vi "Stimulus to 5734 Io Emulator.vi"() -> ()   [LabVIEW 2012]
panel:
  in  "Marker Position":u32
  in  "Frequency":dbl=10000000.0 format="%#_p"
  in  "signal type":T1(ring)
  in  "stop":bool
  out "Data Generated":cluster{"Data":i16, i16}(graph)
  in  "sampling info":cluster{"Fs":dbl, "#s":dbl}={"Fs"=250000000.0, "#s"=1000.0} {"Fs" format="%#_p"}
  # "You cannot change waveform type on the fly"
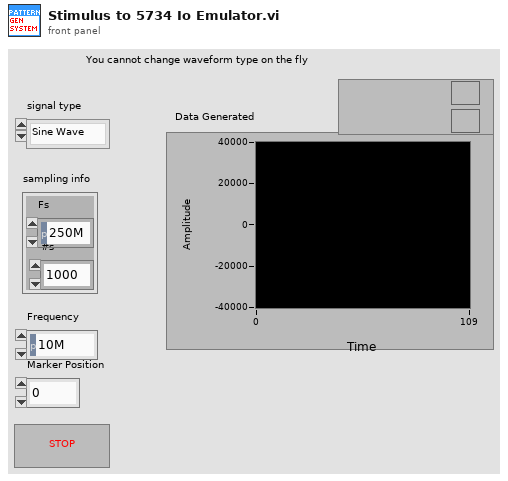
[diagram p1: front panel]
types:
  T1 = enum16{"Sine Wave", "Triangle Wave", "Square Wave", "Sawtooth Wave"}
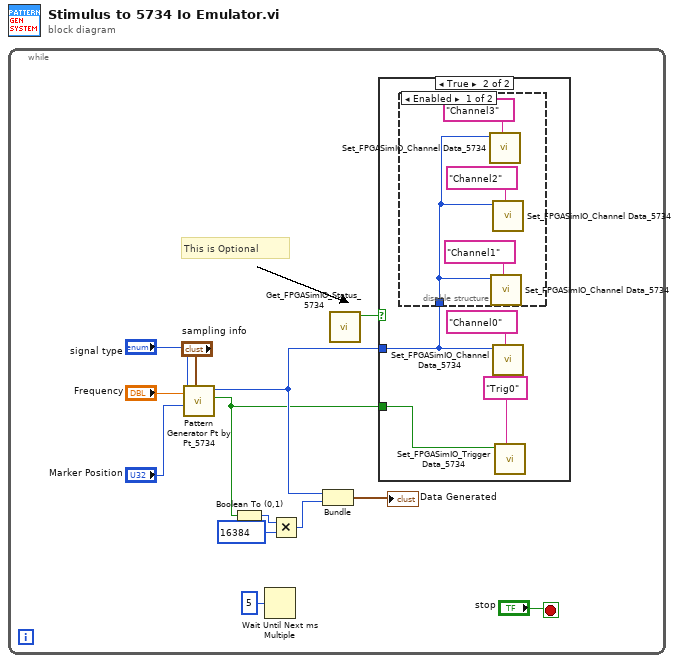
[diagram p0: block diagram]
diagram:
  n1 = while {
    stop <- "stop" stop-if-true
    # "This is Optional"
    n2 = call "Pattern Generator Pt by Pt_5734.vi"("sampling info"="sampling info", "Marker Position"="Marker Position", "signal type"="signal type", "Frequency"="Frequency") -> ("Marker"=w2:bool, "Data"=w3:i16)  [unwired: 4 in, 2 out]
    n3 = Boolean To (0,1)(Boolean=w2) -> (0, 1=w9:i16)
    n4 = Wait Until Next ms Multiple(millisecond multiple=u32 5) -> ()  [unwired: 1 out]
    n5 = Multiply(x=w9, y=i16 16384) -> (x*y=w7:i16)
    n6 = Bundle("Data"=w3, w7) -> (→"Data Generated":cluster{"Data":i16, i16})  [unwired: 1 in]
    n7 = call "Get_FPGASimIO_Status_5734.vi"() -> ("Sim IO FPGA Status"=w1:bool)  [unwired: 10 in, 1 out]
    n8 = case shown="True" w1 {
      tunnel: w3 -> [_ w14]
      tunnel: w2 -> [_ w15]
      frame False {
      }
      frame True {
        n9 = disable-structure shown="Enabled" {
          disable-tunnel: w14 -> [w18 _]
          frame Enabled {
            n10 = call "Set_FPGASimIO_Channel Data_5734.vi"("Channel Name"="Channel3" ("IO Node Name"), "Data"=w18) -> ()  [unwired: 9 in, 1 out]
            n11 = call "Set_FPGASimIO_Channel Data_5734.vi"("Channel Name"="Channel1" ("IO Node Name"), "Data"=w18) -> ()  [unwired: 9 in, 1 out]
            n12 = call "Set_FPGASimIO_Channel Data_5734.vi"("Channel Name"="Channel2" ("IO Node Name"), "Data"=w18) -> ()  [unwired: 9 in, 1 out]
          }
          frame Disabled {
          }
        }
        n13 = call "Set_FPGASimIO_Channel Data_5734.vi"("Channel Name"="Channel0" ("IO Node Name"), "Data"=w14) -> ()  [unwired: 9 in, 1 out]
        n14 = call "Set_FPGASimIO_Trigger Data_5734.vi"("Channel Name"="Trig0" ("IO Node Name"), "Trig Data"=w15) -> ()  [unwired: 9 in, 1 out]
      }
    }
  }
